vi "Add Channels to Task.vi"(0 "task in":refnum<k21>, 5 "channel table":T1[](array[typedef]) {"input terminal configuration" items=["default"=-1, "RSE"=10083, "NRSE"=10078, "Differential"=10106, "Pseudodifferential"=12529]; "Channel Type" items=["Voltage (V)"=0, "Charge (C)"=9, "-"=99, "SPL (Pa)"=3, "Force (lbf)"=6, "Force (N)"=1, "Acceleration (g) - IEPE"=2, "Acceleration (g) - Charge"=12, "Acceleration (g) - 4 wire DC Voltage"=22, "Velocity (in/s)"=7, "Velocity (mm/s)"=8, "Prox Probe (mil)"=4, "Prox Probe (mm)"=5]}, 11 "error in":errorcluster) -> (4 "task out":refnum<k21>, 15 "error out":errorcluster)   [LabVIEW 2024, in "Dynamic Signal Acquisition (Interactive) UI.lvlib"]
uses:
  Dynamic Signal Acquisition (Interactive) UI.lvlib
  SFPDAQmx Channel Info.ctl
  <vilib>/addons/Sound and Vibration/svt_DAQmx/Configuration XControl/Controls/svx_DAQ_Excitation.ctl
  <vilib>/addons/Sound and Vibration/svt_DAQmx/Configuration XControl/Controls/svx_DAQ_ChannelType.ctl
  <resource>/objmgr/daqmx.rc
  <vilib>/addons/Sound and Vibration/svt_DAQmx/Configuration XControl/SVX NI-DAQmx AI Configuration XControl.xctl
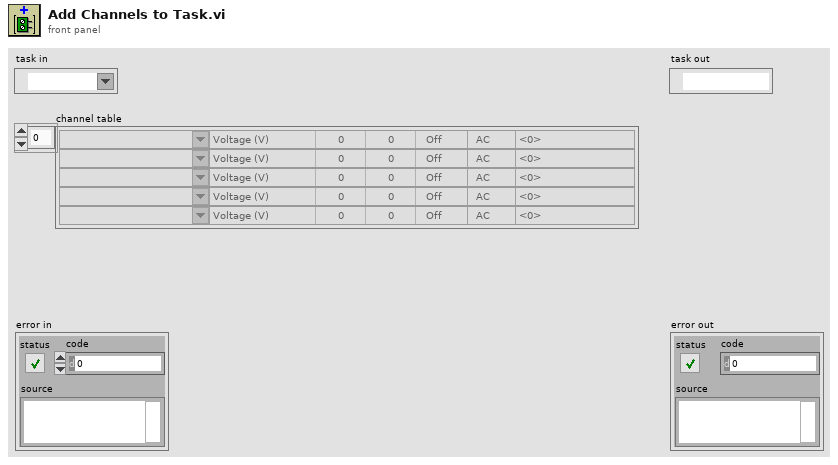
[diagram p1: front panel]
types:
  T1 = typedef "Dynamic Signal Acquisition (Interactive) UI.lvlib/SFPDAQmx Channel Info.ctl" = cluster{"Initialized?":bool, "DAQmx Channel":tag, "Channel Type":u16, "Max":dbl, "Sensitivity":dbl, "Excitation":bool, "Coupling":enum16{"AC", "DC"}, "input terminal configuration":i32, "excitation":enum16{"Off", "Min", "Max"}}
  T2 = typedef "svx_DAQ_Excitation.ctl" = enum16{"Off", "Min", "Max"}
  T3 = typedef "SVX NI-DAQmx AI Configuration XControl.xctl/svx_DAQ_ChannelType.ctl" = u16
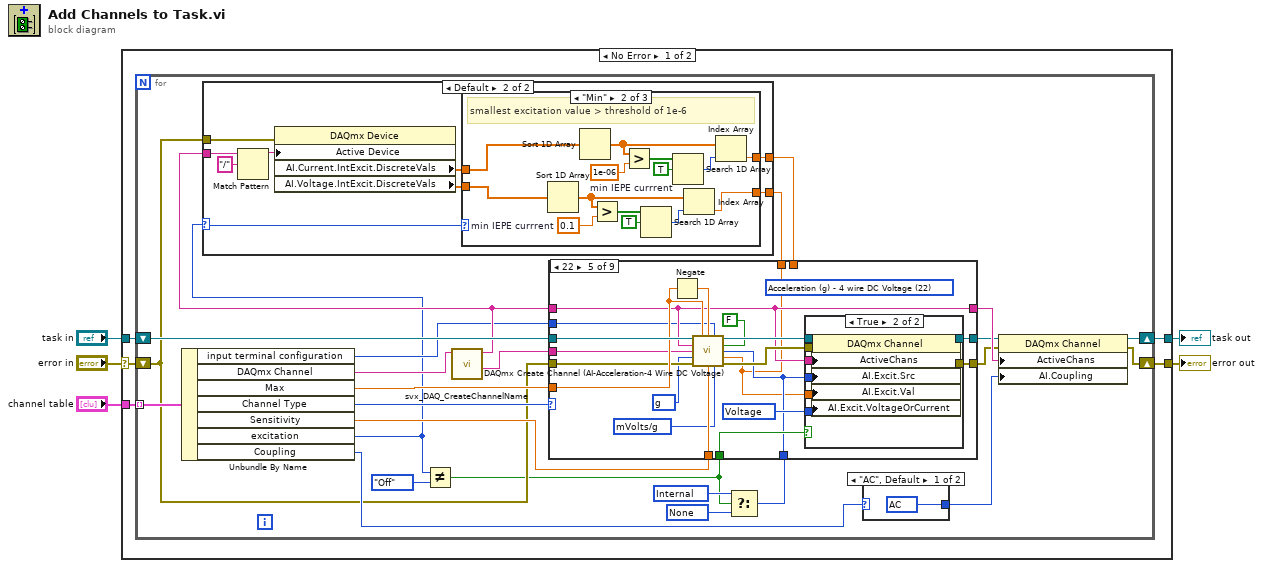
[diagram p0: block diagram]
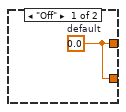
[diagram p2: hidden frame]
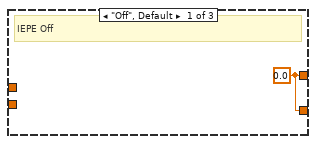
[diagram p3: hidden frame]
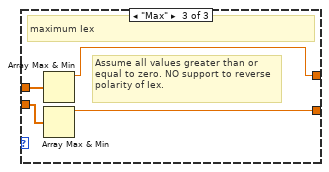
[diagram p4: hidden frame]
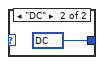
[diagram p5: hidden frame]
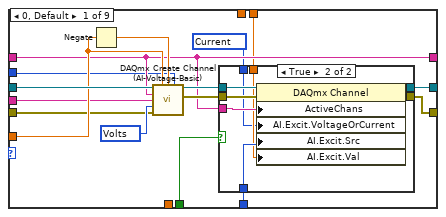
[diagram p6: hidden frame]
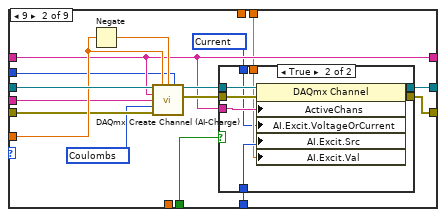
[diagram p8: hidden frame]
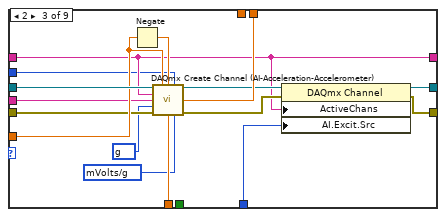
[diagram p10: hidden frame]
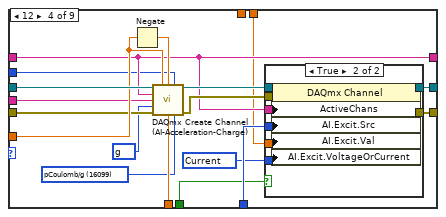
[diagram p11: hidden frame]
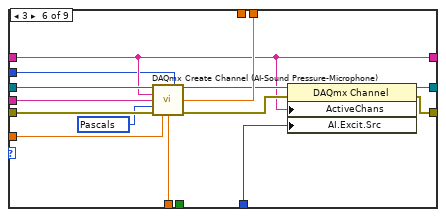
[diagram p14: hidden frame]
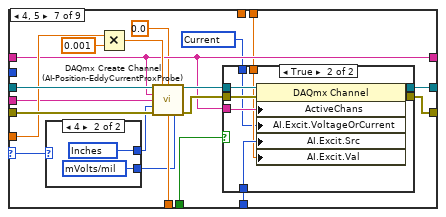
[diagram p15: hidden frame]
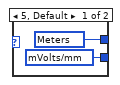
[diagram p16: hidden frame]
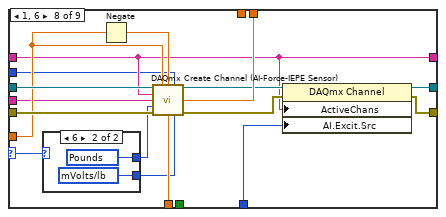
[diagram p18: hidden frame]
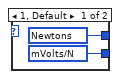
[diagram p19: hidden frame]
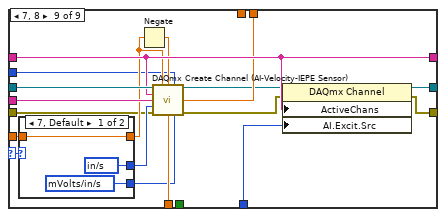
[diagram p20: hidden frame]
diagram:
  n1 = case shown="No Error" "error in" {
    selector: "error in" -> [w7 w287]
    tunnel: "channel table" -> [w10 _]
    tunnel: [w9 w287] -> w4
    tunnel: [w8 w288] -> w3
    tunnel: "task in" -> [w6 w288]
    frame No Error {
      n2 = for {
        tunnel: w10 -> [w34] mode=indexing
        shift-right: [w22] -> w9
        shift-left: w7 -> [w15]
        shift-right: [w23] -> w8
        shift-left: w6 -> [w35]
        w17 = 10230 items=["Internal"=10200, "External"=10167, "None"=10230] ("AI.Excit.Src")
        w18 = 10200 items=["Internal"=10200, "External"=10167, "None"=10230] ("AI.Excit.Src")
        n3 = Unbundle By Name(w34) -> ("input terminal configuration"=w21:i32, "DAQmx Channel"=w29:tag, "Max"=w19:dbl, "Channel Type"=w25:u16, "Sensitivity"=w24:dbl, "excitation"=w11:enum16{"Off", "Min", "Max"}, "Coupling"=w20:enum16{"AC", "DC"})
        n4 = Not Equal?(x=w11, y=svx_DAQ_Excitation."Off") -> (x != y?=w13:bool)
        n5 = call <vilib>:"svx_DAQ_CreateChannelName.vi"("DAQmx Channel In"=w29) -> ("Channel Name"=w26:string, "DAQmx Channel Out"=w27:tag)  [unwired: 9 in]
        n6 = case shown="Default" w11 {
          selector: w11 -> [_ w38]
          tunnel: w15 -> [_ w43]
          tunnel: [w36 w41] -> w28
          tunnel: w27 -> [_ w40]
          tunnel: [w36 w37] -> w12
          frame "Off" {
            w36 = 0.0  # default
          }
          frame Default {
            n7 = Match Pattern(string=w40, regular expression="/") -> (before substring=w44:string)  [unwired: 1 in, 3 out]
            n8 = property class="DAQmx Device"(error in=w43, "Active Device"=w44) -> ("AI.Current.IntExcit.DiscreteVals"=w42:dbl[], "AI.Voltage.IntExcit.DiscreteVals"=w39:dbl[])  [unwired: 1 in, 2 out]
            n9 = case shown="\"Min\"" w38 {
              tunnel: w42 -> [_ w60 w64]
              tunnel: [w46 w59 w63] -> w41
              tunnel: w39 -> [_ w47 w62]
              tunnel: [w46 w48 w61] -> w37
              frame "Off", Default {
                w46 = 0.0
                # "IEPE Off"
              }
              frame "Min" {
                w50 = 0.1  # min IEPE currrent
                w57 = 1e-06  # min IEPE currrent
                # "smallest excitation value > threshold of 1e-6"
                n10 = Sort 1D Array(array=w47) -> (sorted array=w49:dbl[])
                n11 = Sort 1D Array(array=w60) -> (sorted array=w58:dbl[])
                n12 = Greater?(x=w49, y=w50) -> (0:w51:bool[])
                n13 = Greater?(x=w58, y=w57) -> (0:w56:bool[])
                n14 = Search 1D Array(1D array=w51, element=TRUE) -> (index of element=w53:i32)  [unwired: 1 in]
                n15 = Search 1D Array(1D array=w56, element=TRUE) -> (index of element=w54:i32)  [unwired: 1 in]
                n16 = Index Array(array=w49, index=w53) -> (element=w48:dbl)
                n17 = Index Array(array=w58, index=w54) -> (element=w59:dbl)
              }
              frame "Max" {
                # "Assume all values greater than or equal to zero. NO support to reverse polarity of Iex."
                # "maximum Iex"
                n18 = Array Max & Min(array=w64) -> (max value=w63:dbl)  [unwired: 3 out]
                n19 = Array Max & Min(array=w62) -> (max value=w61:dbl)  [unwired: 3 out]
              }
            }
          }
        }
        n20 = Select(t=w18, s=w13, f=w17) -> (s? t:f=w16:i32)
        n21 = case shown="22" w25 {
          selector: w25 -> [_ _ _ _ _ _ w211 w243 w275]
          tunnel: w35 -> [w82 w108 w134 w152 w181 w205 w225 w256 w273]
          tunnel: w27 -> [w72 w99 w124 w143 w172 w196 w216 w246 w272]
          tunnel: w19 -> [w80 w107 w133 w151 w180 w204 w221 w253 w274]
          tunnel: w24 -> [_ _ w129 w147 w176 w202 w223 w254 w267]
          tunnel: w15 -> [w78 w105 w131 w149 w178 w203 w224 w255 w262]
          tunnel: [w75 w102 w122 w140 w170 w199 w215 w250 w278] -> w31
          tunnel: [w74 w101 w123 w141 w171 w194 w214 w249 w277] -> w30
          tunnel: [w72 w99 w124 w143 w172 w196 w216 w246 w272] -> w32
          tunnel: w13 -> [w73 w100 _ w135 w166 _ w219 _ _]
          tunnel: w28 -> [w68 w95 w127 w136 _ w200 w207 w251 w265]
          tunnel: w16 -> [w69 w96 w119 w142 w164 w195 w208 w245 w276]
          tunnel: w26 -> [w71 w98 w121 w139 w169 w193 w212 w244 w271]
          tunnel: w21 -> [w70 w97 w120 w138 w168 w192 _ w240 w261]
          tunnel: w12 -> [_ _ _ _ w163 _ _ _ _]
          frame 0, Default {
            w67 = 10134 items=["Voltage"=10322, "Current"=10134] ("AI.Excit.VoltageOrCurrent")
            w81 = 10348 items=["Volts"=10348, "From Custom Scale"=10065] ("units")
            n22 = Negate(x=w80) -> (-x=w79:dbl)
            n23 = call <vilib>:"DAQmx Create Channel (AI-Voltage-Basic).vi"("task in"=w82, "maximum value"=w80, "minimum value"=w79, "input terminal configuration"=w70, "physical channels"=w72, "name to assign"=w71, "units"=w81, "error in"=w78) -> ("task out"=w77:refnum<k21>, "error out"=w76:errorcluster)  [unwired: 6 in]
            n24 = case shown="True" w73 {
              tunnel: w77 -> [w84 w92]
              tunnel: w76 -> [w83 w91]
              tunnel: w72 -> [_ w90]
              tunnel: [w84 w89] -> w75
              tunnel: [w83 w88] -> w74
              tunnel: w69 -> [_ w87]
              tunnel: w68 -> [_ w86]
              tunnel: w67 -> [_ w85]
              frame False {
              }
              frame True {
                n25 = property class="DAQmx Channel"(reference=w92, error in=w91, "ActiveChans"=w90, "AI.Excit.VoltageOrCurrent"=w85, "AI.Excit.Src"=w87, "AI.Excit.Val"=w86) -> (reference out=w89:refnum<k21>, error out=w88:errorcluster)
              }
            }
          }
          frame 9 {
            w93 = 16102 items=["Coulombs"=16102, "pCoulombs"=16103, "From Custom Scale"=10065] ("units")
            w94 = 10134 items=["Voltage"=10322, "Current"=10134] ("AI.Excit.VoltageOrCurrent")
            n26 = Negate(x=w107) -> (-x=w106:dbl)
            n27 = call <vilib>:"DAQmx Create Channel (AI-Charge).vi"("task in"=w108, "maximum value"=w107, "minimum value"=w106, "input terminal configuration"=w97, "physical channels"=w99, "name to assign"=w98, "units"=w93, "error in"=w105) -> ("task out"=w104:refnum<k21>, "error out"=w103:errorcluster)  [unwired: 6 in]
            n28 = case shown="True" w100 {
              tunnel: w104 -> [w110 w118]
              tunnel: w103 -> [w109 w117]
              tunnel: w99 -> [_ w116]
              tunnel: [w110 w115] -> w102
              tunnel: [w109 w114] -> w101
              tunnel: w96 -> [_ w113]
              tunnel: w95 -> [_ w112]
              tunnel: w94 -> [_ w111]
              frame False {
              }
              frame True {
                n29 = property class="DAQmx Channel"(reference=w118, error in=w117, "ActiveChans"=w116, "AI.Excit.VoltageOrCurrent"=w111, "AI.Excit.Src"=w113, "AI.Excit.Val"=w112) -> (reference out=w115:refnum<k21>, error out=w114:errorcluster)
              }
            }
          }
          frame 2 {
            w128 = 12509 items=["mVolts/g"=12509, "Volts/g"=12510] ("sensitivity units")
            w130 = 10186 items=["g"=10186, "m/s^2"=12470, "From Custom Scale"=10065] ("units")
            n30 = Negate(x=w133) -> (-x=w132:dbl)
            n31 = call <vilib>:"DAQmx Create Channel (AI-Acceleration-Accelerometer).vi"("task in"=w134, "maximum value"=w133, "minimum value"=w132, "input terminal configuration"=w120, "physical channels"=w124, "name to assign"=w121, "current excitation value"=w127, "units"=w130, "error in"=w131, "sensitivity"=w129, "sensitivity units"=w128) -> ("task out"=w126:refnum<k21>, "error out"=w125:errorcluster)  [unwired: 3 in]
            n32 = property class="DAQmx Channel"(reference=w126, error in=w125, "ActiveChans"=w124, "AI.Excit.Src"=w119) -> (reference out=w122:refnum<k21>, error out=w123:errorcluster)
          }
          frame 12 {
            w146 = 16099 items=["pCoulomb/g"=16099, "pCoulomb/(m/s^2)"=16100, "pCoulomb/(in/s^2)"=16101] ("sensitivity units")
            w137 = 10134 items=["Voltage"=10322, "Current"=10134] ("AI.Excit.VoltageOrCurrent")
            w148 = 10186 items=["g"=10186, "m/s^2"=12470, "From Custom Scale"=10065] ("units")
            n33 = Negate(x=w151) -> (-x=w150:dbl)
            n34 = call <vilib>:"DAQmx Create Channel (AI-Acceleration-Charge).vi"("task in"=w152, "maximum value"=w151, "minimum value"=w150, "input terminal configuration"=w138, "physical channels"=w143, "name to assign"=w139, "units"=w148, "error in"=w149, "sensitivity"=w147, "sensitivity units"=w146) -> ("task out"=w145:refnum<k21>, "error out"=w144:errorcluster)  [unwired: 4 in]
            n35 = case shown="True" w135 {
              tunnel: w145 -> [w153 w162]
              tunnel: w144 -> [w154 w161]
              tunnel: w143 -> [_ w160]
              tunnel: w142 -> [_ w159]
              tunnel: [w154 w158] -> w141
              tunnel: [w153 w157] -> w140
              tunnel: w137 -> [_ w156]
              tunnel: w136 -> [_ w155]
              frame False {
              }
              frame True {
                n36 = property class="DAQmx Channel"(reference=w162, error in=w161, "ActiveChans"=w160, "AI.Excit.Src"=w159, "AI.Excit.Val"=w155, "AI.Excit.VoltageOrCurrent"=w156) -> (reference out=w157:refnum<k21>, error out=w158:errorcluster)
              }
            }
          }
          frame 22 {
            (unwired) T3 22 items=["Voltage (V)"=0, "Charge (C)"=9, "-"=99, "SPL (Pa)"=3, "Force (lbf)"=6, "Force (N)"=1, "Acceleration (g) - IEPE"=2, "Acceleration (g) - Charge"=12, "Acceleration (g) - 4 wire DC Voltage"=22, "Velocity (in/s)"=7, "Velocity (mm/s)"=8, "Prox Probe (mil)"=4, "Prox Probe (mm)"=5] ("Channel Type")
            w175 = 12509 items=["mVolts/g"=12509, "Volts/g"=12510] ("sensitivity units")
            w167 = 10322 items=["Voltage"=10322, "Current"=10134] ("AI.Excit.VoltageOrCurrent")
            w177 = 10186 items=["g"=10186, "m/s^2"=12470, "From Custom Scale"=10065] ("units")
            n37 = Negate(x=w180) -> (-x=w179:dbl)
            n38 = call <vilib>:"DAQmx Create Channel (AI-Acceleration-4 Wire DC Voltage).vi"("task in"=w181, "maximum value"=w180, "minimum value"=w179, "input terminal configuration"=w168, "physical channels"=w172, "use excitation for scaling"=FALSE, "name to assign"=w169, "voltage excitation source"=w164, "units"=w177, "voltage excitation value"=w163, "error in"=w178, "sensitivity"=w176, "sensitivity units"=w175) -> ("task out"=w174:refnum<k21>, "error out"=w173:errorcluster)  [unwired: 1 in]
            n39 = case shown="True" w166 {
              tunnel: w174 -> [w182 w191]
              tunnel: w173 -> [w183 w190]
              tunnel: w172 -> [_ w189]
              tunnel: w164 -> [_ w188]
              tunnel: [w183 w187] -> w171
              tunnel: [w182 w186] -> w170
              tunnel: w167 -> [_ w185]
              tunnel: w163 -> [_ w184]
              frame False {
              }
              frame True {
                n40 = property class="DAQmx Channel"(reference=w191, error in=w190, "ActiveChans"=w189, "AI.Excit.Src"=w188, "AI.Excit.Val"=w184, "AI.Excit.VoltageOrCurrent"=w185) -> (reference out=w186:refnum<k21>, error out=w187:errorcluster)
              }
            }
          }
          frame 3 {
            w201 = 10081 items=["Pascals"=10081, "From Custom Scale"=10065] ("units")
            n41 = call <vilib>:"DAQmx Create Channel (AI-Sound Pressure-Microphone).vi"("task in"=w205, "maximum sound pressure level"=w204, "input terminal configuration"=w192, "physical channels"=w196, "name to assign"=w193, "current excitation value"=w200, "units"=w201, "error in"=w203, "microphone sensitivity"=w202) -> ("task out"=w198:refnum<k21>, "error out"=w197:errorcluster)  [unwired: 5 in]
            n42 = property class="DAQmx Channel"(reference=w198, error in=w197, "ActiveChans"=w196, "AI.Excit.Src"=w195) -> (reference out=w199:refnum<k21>, error out=w194:errorcluster)
          }
          frame 4, 5 {
            w206 = 10134 items=["Voltage"=10322, "Current"=10134] ("AI.Excit.VoltageOrCurrent")
            n43 = case shown="4" w211 {
              tunnel: [w227 w229] -> w210
              tunnel: [w226 w228] -> w209
              frame 5, Default {
                w226 = 14838 items=["mVolts/mil"=14836, "Volts/mil"=14837, "mVolts/mm"=14838, "Volts/mm"=14839, "mVolts/micron"=14840] ("sensitivity units")
                w227 = 10219 items=["Meters"=10219, "Inches"=10379, "From Custom Scale"=10065] ("units")
              }
              frame 4 {
                w228 = 14836 items=["mVolts/mil"=14836, "Volts/mil"=14837, "mVolts/mm"=14838, "Volts/mm"=14839, "mVolts/micron"=14840] ("sensitivity units")
                w229 = 10379 items=["Meters"=10219, "Inches"=10379, "From Custom Scale"=10065] ("units")
              }
            }
            n44 = Multiply(x=w221, y=0.001) -> (x*y=w220:dbl)
            n45 = call <vilib>:"DAQmx Create Channel (AI-Position-EddyCurrentProxProbe).vi"("task in"=w225, "maximum value"=w220, "minimum value"=0.0, "physical channels"=w216, "name to assign"=w212, "units"=w210, "error in"=w224, "sensitivity"=w223, "sensitivity units"=w209) -> ("task out"=w217:refnum<k21>, "error out"=w218:errorcluster)  [unwired: 5 in]
            n46 = case shown="True" w219 {
              tunnel: w217 -> [w231 w239]
              tunnel: w218 -> [w230 w238]
              tunnel: w216 -> [_ w237]
              tunnel: [w231 w236] -> w215
              tunnel: [w230 w235] -> w214
              tunnel: w208 -> [_ w234]
              tunnel: w207 -> [_ w233]
              tunnel: w206 -> [_ w232]
              frame False {
              }
              frame True {
                n47 = property class="DAQmx Channel"(reference=w239, error in=w238, "ActiveChans"=w237, "AI.Excit.VoltageOrCurrent"=w232, "AI.Excit.Src"=w234, "AI.Excit.Val"=w233) -> (reference out=w236:refnum<k21>, error out=w235:errorcluster)
              }
            }
          }
          frame 1, 6 {
            n48 = case shown="6" w243 {
              tunnel: [w258 w260] -> w242
              tunnel: [w257 w259] -> w241
              frame 1, Default {
                w257 = 15891 items=["mVolts/N"=15891, "mVolts/lb"=15892] ("sensitivity units")
                w258 = 15875 items=["Newtons"=15875, "Pounds"=15876, "kgf"=15877, "From Custom Scale"=10065] ("units")
              }
              frame 6 {
                w259 = 15892 items=["mVolts/N"=15891, "mVolts/lb"=15892] ("sensitivity units")
                w260 = 15876 items=["Newtons"=15875, "Pounds"=15876, "kgf"=15877, "From Custom Scale"=10065] ("units")
              }
            }
            n49 = Negate(x=w253) -> (-x=w252:dbl)
            n50 = call <vilib>:"DAQmx Create Channel (AI-Force-IEPE Sensor).vi"("task in"=w256, "maximum value"=w253, "minimum value"=w252, "input terminal configuration"=w240, "physical channels"=w246, "name to assign"=w244, "current excitation value"=w251, "units"=w242, "error in"=w255, "sensitivity"=w254, "sensitivity units"=w241) -> ("task out"=w248:refnum<k21>, "error out"=w247:errorcluster)  [unwired: 3 in]
            n51 = property class="DAQmx Channel"(reference=w248, error in=w247, "ActiveChans"=w246, "AI.Excit.Src"=w245) -> (reference out=w250:refnum<k21>, error out=w249:errorcluster)
          }
          frame 7, 8 {
            n52 = case shown="7, Default" w275 {
              tunnel: [w281 w286] -> w268
              tunnel: [w280 w285] -> w266
              tunnel: w274 -> [w279 w283]
              tunnel: [w279 w282] -> w269
              frame 7, Default {
                w280 = 15964 items=["mVolts/mm/s"=15963, "mVolts/in/s"=15964] ("sensitivity units")
                w281 = 15960 items=["m/s"=15959, "in/s"=15960, "From Custom Scale"=10065] ("units")
              }
              frame 8 {
                w285 = 15963 items=["mVolts/mm/s"=15963, "mVolts/in/s"=15964] ("sensitivity units")
                w286 = 15959 items=["m/s"=15959, "in/s"=15960, "From Custom Scale"=10065] ("units")
                n53 = Multiply(x=w283, y=0.001) -> (x*y=w282:dbl)
              }
            }
            n54 = Negate(x=w269) -> (-x=w270:dbl)
            n55 = call <vilib>:"DAQmx Create Channel (AI-Velocity-IEPE Sensor).vi"("task in"=w273, "maximum value"=w269, "minimum value"=w270, "input terminal configuration"=w261, "physical channels"=w272, "name to assign"=w271, "current excitation value"=w265, "units"=w268, "error in"=w262, "sensitivity"=w267, "sensitivity units"=w266) -> ("task out"=w264:refnum<k21>, "error out"=w263:errorcluster)  [unwired: 3 in]
            n56 = property class="DAQmx Channel"(reference=w264, error in=w263, "ActiveChans"=w272, "AI.Excit.Src"=w276) -> (reference out=w278:refnum<k21>, error out=w277:errorcluster)
          }
        }
        n57 = case shown="\"AC\", Default" w20 {
          tunnel: [w65 w66] -> w33
          frame "AC", Default {
            w65 = 10045 items=["AC"=10045, "DC"=10050, "GND"=10066] ("AI.Coupling")
          }
          frame "DC" {
            w66 = 10050 items=["AC"=10045, "DC"=10050, "GND"=10066] ("AI.Coupling")
          }
        }
        n58 = property class="DAQmx Channel"(reference=w31, error in=w30, "ActiveChans"=w32, "AI.Coupling"=w33) -> (reference out=w23:refnum<k21>, error out=w22:errorcluster)
      }
    }
    frame Error {
    }
  }
  "error out" <- w4
  "task out" <- w3
